vi "ArchViewer.vi"() -> ()   [LabVIEW 2010]
doc: "Use this template to create an application that executes until you click the Stop button. Unlike the Single Loop Application VI that uses polling, this VI uses the Event structure."
uses:
  <vilib>/addons/database/Connection.llb/DB Tools Open Connec (Path).vi
  <vilib>/addons/database/NI_Database_API.lvlib
panel:
  in  "save":bool
  out "Message":string
  out "ObjProp":string[][](table)
  in  "ViewMode":enum32{"Графики", "Тренды/Отчет", "SQL"}(tab)=enum."Тренды/Отчет"
  out "phwnd":string[][](table)
  out "reason":string caption="Описание"
  in  "DateAndTime":u16(ring) caption="Дата и Время" items=["2012-04-04 23:22:02", "2012-05-04 20:10:38"]
  out "Waveform Graph":cluster{sgl, sgl, sgl[]}[](graph)
  in  "CurvesName":i32(ring) caption="Сигнал (Тип сигнала)" items=["Q(wt)max"=400301, "Q(wt)mean"=500301, "Q(R)"=300301, "I(R)"=100301, "N(Q)"=200301]
  in  "DateAndTime 2":u16(ring) caption="Дата и Время" items=["2012-04-04 23:22:02", "2012-05-04 20:10:38"]
  in  "Создать отчет":bool
  out "XY Graph":cluster{timestamp[], sgl[]}(graph)
  in  "T final":timestamp caption="Конец интервала"
  in  "T start":timestamp caption="Начало"
  in  "SigName":u16(ring) caption="Сигнал" items=["Ch1(I(R=0,5))"=2, "Ch1(Q(R=0,5))"=1, "Ch2(I(R=0,5))"=4, "Ch2(Q(R=0,5))"=3, "Ch3(I(R=0,5))"=6, "Ch3(Q(R=0,5))"=5, "Ch4(I(R=0,5))"=8, "Ch4(Q(R=0,5))"=7, "In(Напряжение/Ток)"=10, "In(Частота)"=11, "Out(Напряжение/Ток)"=9]
  in  "Numeric":i32 min=0 max=9
  in  "Execute":bool
  out "Data":string[][](table) caption="Данные"
  in  "Query":string caption="Запрос"
  in  "Tables":i32(listbox) caption="Таблицы"
  in  "Object":u16(ring) caption="Объект" items=["К-19 Тц", "xz_name", "test_5", "object", "object", "xz_name", "object"]
  in  "stop":bool
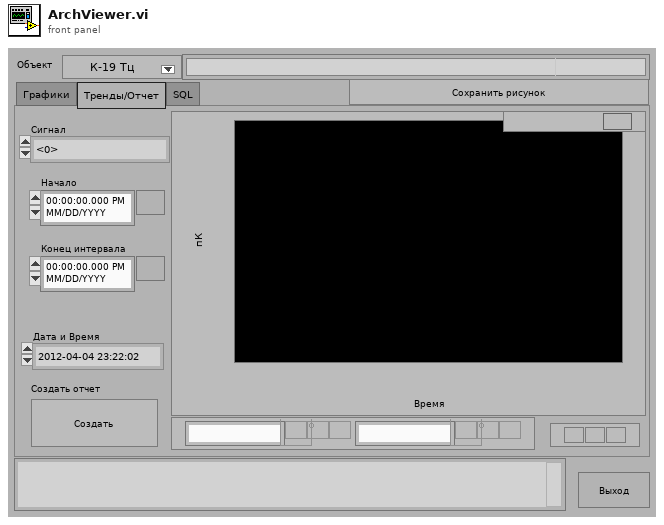
[diagram p1: front panel]
types:
  T1 = cluster{"Number":string, "Obj":string, "SerNum":string, "Graphs":cluster{"Numeric":dbl, "Time Stamp":timestamp, "Array":dbl[]}[]}
  T2 = typedef "NI_Database_API.lvlib/Conn ObjectReference.ctl" = refnum<k1>
  T3 = cluster{"recordset data[0]":variant, "recordset data[1]":variant}
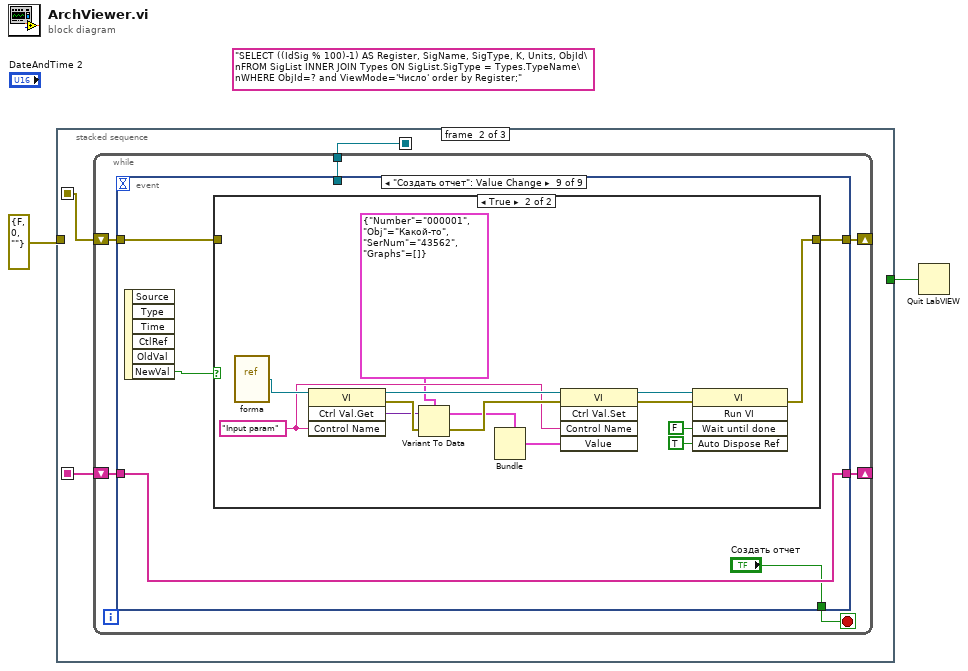
[diagram p0: block diagram]
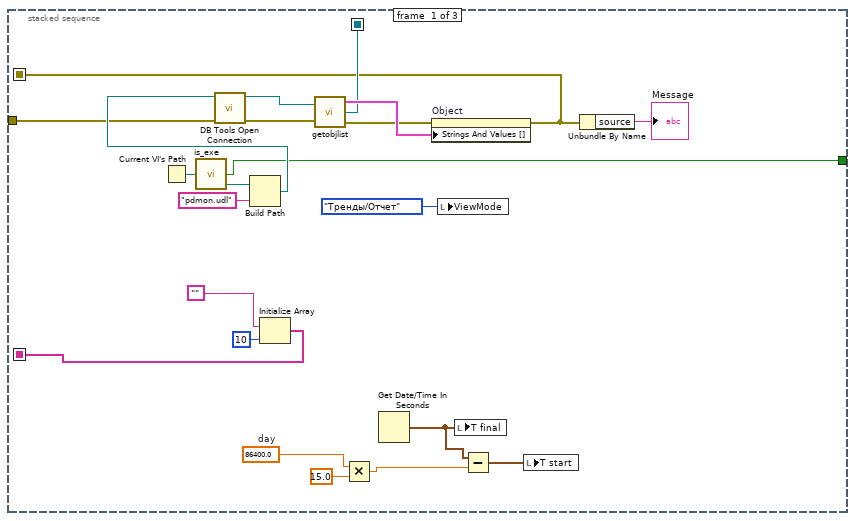
[diagram p2: hidden frame]
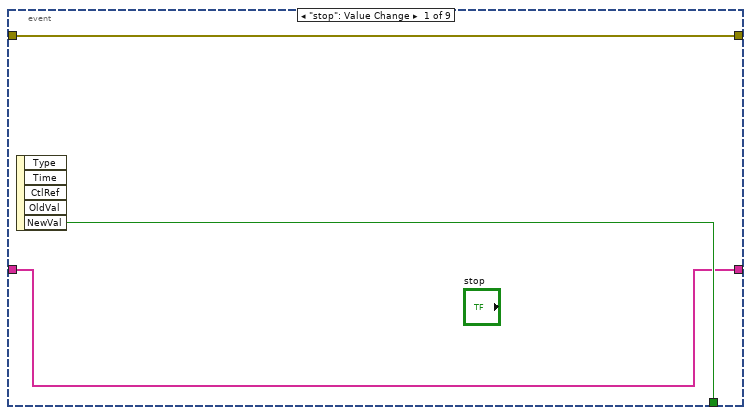
[diagram p3: hidden frame]
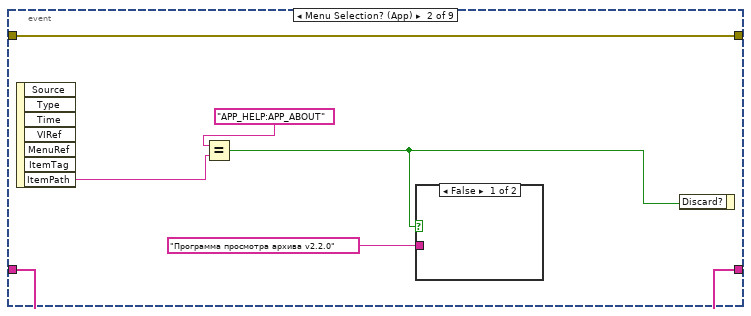
[diagram p4: hidden frame]
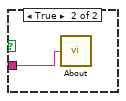
[diagram p5: hidden frame]
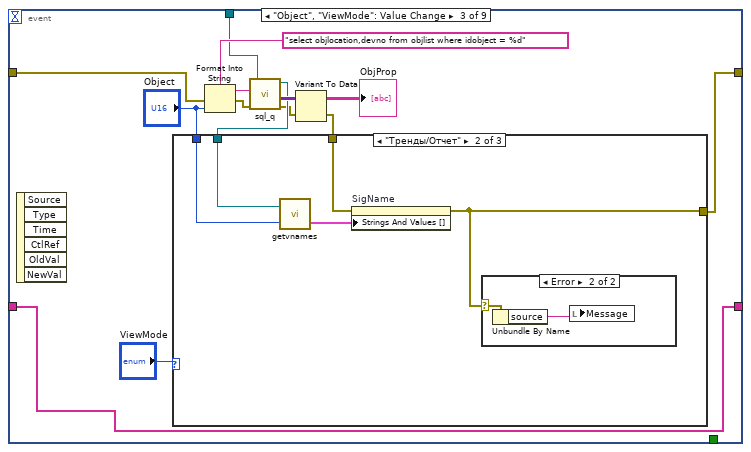
[diagram p6: hidden frame]
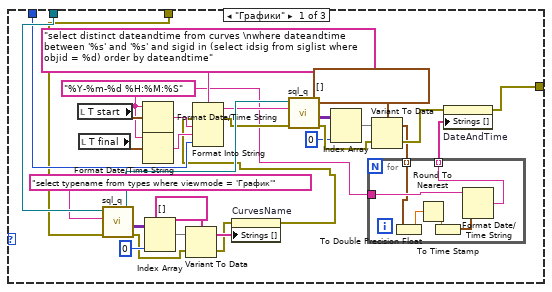
[diagram p7: hidden frame]
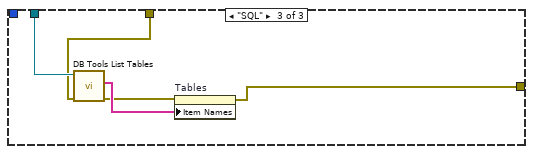
[diagram p9: hidden frame]
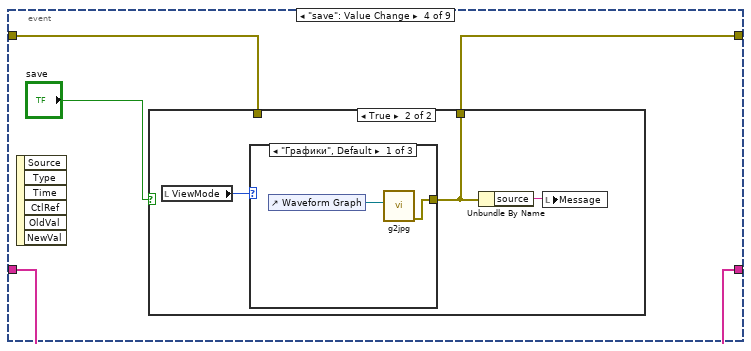
[diagram p10: hidden frame]
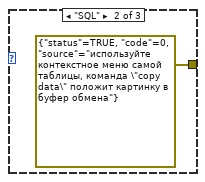
[diagram p12: hidden frame]
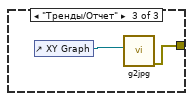
[diagram p13: hidden frame]
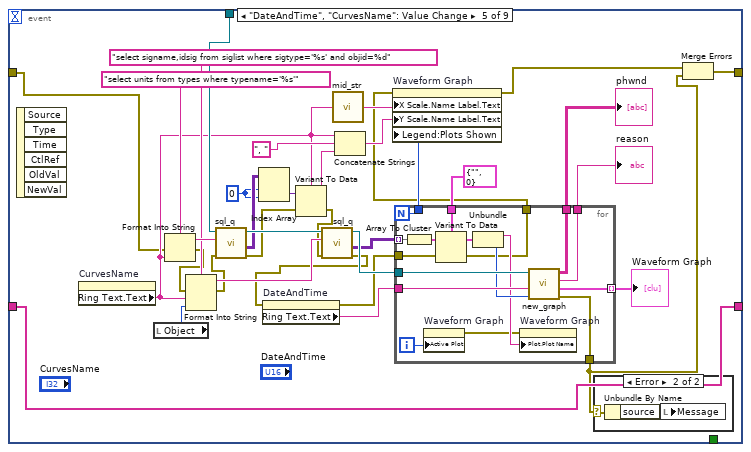
[diagram p14: hidden frame]
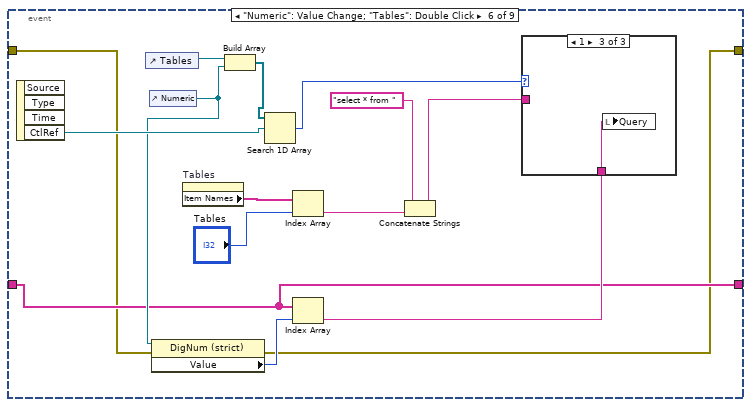
[diagram p16: hidden frame]
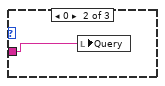
[diagram p18: hidden frame]
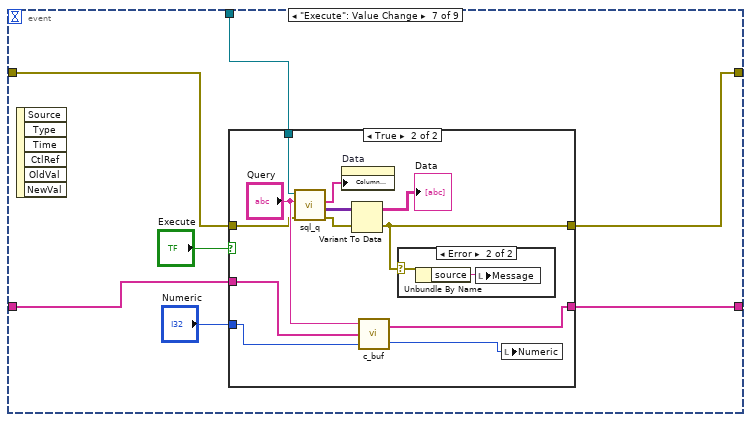
[diagram p19: hidden frame]
diagram:
  (unwired) "SELECT ((IdSig % 100)-1) AS Register, SigName, SigType, K, Units, ObjId\nFROM SigList INNER JOIN Types ON SigList.SigType = Types.TypeName\nWHERE ObjId=? and ViewMode='Число' order by Register;"
  n1 = stacked-sequence {
    seq-local: [w20 _ _] -> [_ w27 w248]
    seq-local: [w7 _ _] -> [_ w26 _]
    seq-local: [w3 _ _] -> [_ w25 _]
    tunnel: [w6 _ _] -> w2
    tunnel: errorcluster {"status"=FALSE, "code"=0, "source"=""} ("error out") -> [w4 _ _]
    frame #0 {
      w12 = 86400.0  # day
      n2 = Current VI's Path() -> (path=w18:path)
      n3 = call "is_exe.vi"("path"=w18) -> ("actual path"=w17:path, "exe?"=w6:bool)  [unwired: 2 in, 1 out]
      n4 = Build Path(base path=w17, name or relative path="pdmon.udl") -> (appended path=w15:path)
      n5 = call-poly <vilib>:"DB Tools Open Connection.vi"("error in (no error)"=w4, "connection information"=w15) -> ("error out"=w21:errorcluster, "connection reference"=w22:T2)  [unwired: 6 in]
      n6 = Initialize Array("", 10 ("dimension size")) -> (w7:string[])
      n7 = call "getobjlist.vi"("connection"=w22, "error in"=w21) -> ("StringsAndValues[]"=w24:cluster{"String":string, "Value":u16}[], "connection out"=w20:T2, "error out"=w23:errorcluster)
      n8 = Multiply(x=w12, y=15.0) -> (x*y=w11:dbl)
      n9 = Get Date/Time In Seconds() -> (seconds since 1Jan1904=w14:timestamp)
      n10 = property on="Object" class="Ring (strict)"(error in=w23, "Strings And Values []"=w24) -> (error out=w3:errorcluster)  [unwired: 1 in, 1 out]
      n11 = local write "ViewMode"(enum32{"Графики", "Тренды/Отчет", "SQL"}."Тренды/Отчет" ("ViewMode")) -> ()
      n12 = local write "T final"(w14) -> ()
      n13 = Subtract(x=w14, y=w11) -> (x-y=w13:timestamp)
      n14 = local write "T start"(w13) -> ()
      n15 = Unbundle By Name(w3) -> ("source"=→"Message":string)
    }
    frame #1 {
      n16 = while {
        tunnel: w27 -> [w32]
        shift-right: [w31] -> _
        shift-left: w26 -> [w30]
        shift-right: [w28] -> _
        shift-left: w25 -> [w29]
        stop <- w33 stop-if-true
        n17 = event shown="[8] \"Создать отчет\": Value Change" {
          selector: _ -> [_ _ _ _ _ _ _ _ _]
          dyn-events: _ -> [_ _ _ _ _ _ _ _ _]
          timeout: _ -> [_ _ _ _ _ _ _ _ _]
          tunnel: [w36 _ _ _ _ _ _ _ "Создать отчет"] -> w33
          tunnel: w32 -> [_ _ w53 _ w142 _ w196 w225 _]
          tunnel: [w35 w42 w47 w108 w130 w175 w193 w218 w232] -> w31
          tunnel: w30 -> [w35 w42 w47 w108 w130 w175 w192 w218 w232]
          tunnel: w29 -> [w34 w37 w46 w106 w126 w174 w191 w216 w231]
          tunnel: [w34 w37 w44 w107 w121 w173 w190 w215 w230] -> w28
          event "stop": Value Change {
            n18 = event-data() -> ("NewVal"=w36:bool)  [unwired: 1 in, 4 out]
          }
          event Menu Selection? (App) {
            n19 = event-data() -> ("ItemPath"=w40:string)  [unwired: 1 in, 6 out]
            n20 = Equal?(x="APP_HELP:APP_ABOUT", y=w40) -> (x = y?=w39:bool)
            n21 = case shown="False" w39 {
              tunnel: "Программа просмотра архива v2.2.0" -> [_ w43]
              frame False {
              }
              frame True {
                n22 = call "About.vi"("Revision Number"=w43) -> ()
              }
            }
            n23 = event-data("Discard?"=w39) -> ()  [unwired: 1 in, 1 out]
          }
          event "Object", "ViewMode": Value Change {
            n24 = event-data() -> ()  [unwired: 1 in, 6 out]
            n25 = Format Into String(format string="select objlocation,devno from objlist where idobject = %d", error in=w46, "Object") -> (resulting string=w56:string, error out=w49:errorcluster)  [unwired: 1 in]
            n26 = call "sql_q.vi"("error in"=w49, "SQL query"=w56, "connect ref"=w53) -> ("error out"=w51:errorcluster, "recordset data"=w55:variant[][], "conn ref out"=w52:T2)  [unwired: 1 in, 1 out]
            n27 = Variant To Data(error in=w51, Variant=w55) -> (error out=w45:errorcluster, data=→"ObjProp":string[][])  [unwired: 1 in]
            n28 = case shown="\"Тренды/Отчет\"" "ViewMode" {
              tunnel: w52 -> [w87 w97 w105]
              tunnel: "Object" -> [w61 w96 _]
              tunnel: w45 -> [w60 w95 w102]
              tunnel: [w58 w94 w101] -> w44
              frame "Графики" {
                w63 = "%Y-%m-%d %H:%M:%S" ("time format string (%c)")
                n29 = local read "T start"() -> (w75:timestamp)
                n30 = local read "T final"() -> (w74:timestamp)
                n31 = call "sql_q.vi"("error in"=w60, "SQL query"="select typename from types where viewmode = 'График'", "connect ref"=w87) -> ("error out"=w80:errorcluster, "recordset data"=w85:variant[][], "conn ref out"=w69:T2)  [unwired: 1 in, 1 out]
                n32 = Format Date/Time String(time format string (%c)=w63, seconds (now)=w75) -> (date/time string=w77:string)  [unwired: 1 in]
                n33 = Format Date/Time String(time format string (%c)=w63, seconds (now)=w74) -> (date/time string=w78:string)  [unwired: 1 in]
                n34 = Index Array(array=w85, index (col)=0 ("disabled index (col)")) -> (element=w82:variant[])  [unwired: 1 in]
                n35 = Variant To Data(error in=w80, Variant=w82, type=string[] [] ("Strings []")) -> (error out=w79:errorcluster, data=w84:string[])
                n36 = property on="CurvesName" class="Ring (strict)"(error in=w79, "Strings []"=w84) -> (error out=w59:errorcluster)  [unwired: 1 in, 1 out]
                n37 = Format Into String(format string="select distinct dateandtime from curves \nwhere dateandtime between '%s' and '%s' and sigid in (select idsig from siglist where objid = %d) order by dateandtime", error in=w59, w77, w78, w61) -> (resulting string=w68:string, error out=w67:errorcluster)  [unwired: 1 in]
                n38 = call "sql_q.vi"("error in"=w67, "SQL query"=w68, "connect ref"=w69) -> ("error out"=w73:errorcluster, "recordset data"=w70:variant[][])  [unwired: 1 in, 2 out]
                n39 = Index Array(array=w70, index (col)=0 ("disabled index (col)")) -> (element=w71:variant[])  [unwired: 1 in]
                n40 = Variant To Data(error in=w73, Variant=w71, type=timestamp[] [] ("Strings []")) -> (error out=w66:errorcluster, data=w65:timestamp[])
                n41 = for {
                  tunnel: w65 -> [w88] mode=indexing
                  tunnel: [w93] -> w64 mode=indexing
                  tunnel: w63 -> [w92]
                  n42 = To Double Precision Float(number=w88) -> (double precision float=w90:dbl)
                  n43 = Round To Nearest(number=w90) -> (nearest integer value=w89:dbl)
                  n44 = To Time Stamp(1:w89) -> (0:w91:timestamp)
                  n45 = Format Date/Time String(time format string (%c)=w92, seconds (now)=w91) -> (date/time string=w93:string)  [unwired: 1 in]
                }
                n46 = property on="DateAndTime" class="Ring (strict)"(error in=w66, "Strings []"=w64) -> (error out=w58:errorcluster)  [unwired: 1 in, 1 out]
              }
              frame "Тренды/Отчет" {
                n47 = call "getvnames.vi"("Object"=w96, "connection reference in"=w97) -> ("StringsAndValues[]"=w98:cluster{"String":string, "Value":u16}[])  [unwired: 1 out]
                n48 = property on="SigName" class="Ring (strict)"(error in=w95, "Strings And Values []"=w98) -> (error out=w94:errorcluster)  [unwired: 1 in, 1 out]
                n49 = case shown="Error" w94 {
                  selector: w94 -> [_ w100]
                  frame No Error {
                  }
                  frame Error {
                    n50 = Unbundle By Name(w100) -> ("source"=w99:string)
                    n51 = local write "Message"(w99) -> ()
                  }
                }
              }
              frame "SQL" {
                n52 = call <vilib>:"DB Tools List Tables.vi"("error in (no error)"=w102, "connection reference"=w105) -> ("error out"=w103:errorcluster, "tables"=w104:string[])  [unwired: 3 in, 1 out]
                n53 = property on="Tables" class="LstBox (strict)"(error in=w103, "Item Names"=w104) -> (error out=w101:errorcluster)  [unwired: 1 in, 1 out]
              }
            }
          }
          event "save": Value Change {
            n54 = event-data() -> ()  [unwired: 1 in, 6 out]
            n55 = case shown="True" "save" {
              tunnel: [w110 w111] -> w107
              tunnel: w106 -> [w110 _]
              frame False {
              }
              frame True {
                n56 = local read "ViewMode"() -> (w113:enum32{"Графики", "Тренды/Отчет", "SQL"})
                n57 = case shown="\"Графики\", Default" w113 {
                  tunnel: [w114 errorcluster {"status"=TRUE, "code"=0, "source"="используйте контекстное меню самой таблицы, команда \"copy data\" положит картинку в буфер обмена"} ("error out") w117] -> w111
                  frame "Графики", Default {
                    n58 = control-ref of="Waveform Graph"() -> (w115:refnum<vi>)
                    n59 = call "g2jpg.vi"("WG"=w115) -> ("error out"=w114:errorcluster)  [unwired: 5 in, 1 out]
                  }
                  frame "SQL" {
                  }
                  frame "Тренды/Отчет" {
                    n60 = control-ref of="XY Graph"() -> (w118:refnum<vi>)
                    n61 = call "g2jpg.vi"("WG"=w118) -> ("error out"=w117:errorcluster)  [unwired: 5 in, 1 out]
                  }
                }
                n62 = Unbundle By Name(w111) -> ("source"=w112:string)
                n63 = local write "Message"(w112) -> ()
              }
            }
          }
          event "DateAndTime", "CurvesName": Value Change {
            w139 = 0
            n64 = event-data() -> ()  [unwired: 1 in, 6 out]
            n65 = property on="CurvesName" class="Ring (strict)"() -> ("Ring Text.Text"=w131:string)  [unwired: 2 in, 2 out]
            n66 = local read "Object"() -> (w150:u16)
            n67 = Format Into String(format string="select units from types where typename='%s'", error in=w126, w131) -> (resulting string=w143:string, error out=w127:errorcluster)  [unwired: 1 in]
            n68 = Format Into String(format string="select signame,idsig from siglist where sigtype='%s' and objid=%d" ("regular expression (\"\")"), error in=w127, w131, w150) -> (resulting string=w151:string, error out=w128:errorcluster)  [unwired: 1 in]
            n69 = call "sql_q.vi"("error in"=w128, "SQL query"=w143, "connect ref"=w142) -> ("error out"=w136:errorcluster, "recordset data"=w140:variant[][], "conn ref out"=w141:T2)  [unwired: 1 in, 1 out]
            n70 = Index Array(array=w140, index (row)=w139, index (col)=w139) -> (element=w138:variant)
            n71 = Variant To Data(error in=w136, Variant=w138, type=w131) -> (error out=w125:errorcluster, data=w135:string)
            n72 = call "sql_q.vi"("error in"=w125, "SQL query"=w151, "connect ref"=w141) -> ("error out"=w120:errorcluster, "recordset data"=w148:variant[][], "conn ref out"=w149:T2)  [unwired: 1 in, 1 out]
            n73 = property on="DateAndTime" class="Ring (strict)"(error in=w120) -> (error out=w119:errorcluster, "Ring Text.Text"=w153:string)  [unwired: 1 in, 1 out]
            n74 = call "mid_str.vi"("String"=w131) -> ("mid substring"=w132:string)  [unwired: 4 in]
            n75 = Concatenate Strings(w131, ", ", w135) -> (w134:string)
            n76 = for {
              N -> [w157]
              tunnel: w153 -> [w170]
              tunnel: [w169] -> w122
              tunnel: [w168] -> w152
              tunnel: w149 -> [w167]
              tunnel: w148 -> [w166] mode=indexing
              tunnel: cluster{string, i32} {"", 0} -> [w165]
              tunnel: [w161] -> w146 mode=indexing
              tunnel: [w157] -> w145
              tunnel: w119 -> [w156]
              tunnel: [w155] -> w124
              tunnel: [w154] -> w129
              i -> [w160]
              n77 = Array To Cluster(array=w166) -> (cluster=w164:T3)
              n78 = property on="Waveform Graph" class="WFGraph (strict)"("Active Plot"=w160) -> (error out=w158:errorcluster)  [unwired: 2 in, 1 out]
              n79 = Variant To Data(error in=w156, Variant=w164, type=w165) -> (error out=w155:errorcluster, data=w163:cluster{string, i32})
              n80 = Unbundle(w163) -> (w159:string, w162:i32)
              n81 = property on="Waveform Graph" class="WFGraph (strict)"(error in=w158, "Plot.Plot Name"=w159) -> ()  [unwired: 1 in, 2 out]
              n82 = call "new_graph.vi"("CurvesId"=w162, "D&T"=w170, "connection ref"=w167) -> ("error out"=w169:errorcluster, "Waveform Graph"=w161:cluster{sgl, sgl, sgl[]}, "reason"=w168:string, "phwnd"=w154:string[][])  [unwired: 1 in]
            }
            "Waveform Graph" <- w146
            "reason" <- w152
            "phwnd" <- w129
            n83 = property on="Waveform Graph" class="WFGraph (strict)"(error in=w124, "X Scale.Name Label.Text"=w132, "Y Scale.Name Label.Text"=w134, "Legend:Plots Shown"=w145) -> (error out=w123:errorcluster)  [unwired: 1 in, 1 out]
            n84 = case shown="Error" w122 {
              selector: w122 -> [_ w172]
              frame No Error {
              }
              frame Error {
                n85 = Unbundle By Name(w172) -> ("source"=w171:string)
                n86 = local write "Message"(w171) -> ()
              }
            }
            n87 = Merge Errors(w123, w122) -> (w121:errorcluster)
          }
          event "Numeric": Value Change; "Tables": Double Click {
            n88 = event-data() -> ("CtlRef"=w181:refnum<vi>)  [unwired: 1 in, 3 out]
            n89 = control-ref of="Tables"() -> (w183:refnum<vi>)
            n90 = control-ref of="Numeric"() -> (w177:refnum<vi>)
            n91 = property on="Property Node" class="DigNum (strict)"(reference=w177, error in=w174) -> (error out=w173:errorcluster, "Value"=w176:i32)  [unwired: 1 out]
            n92 = property on="Tables" class="LstBox (strict)"() -> ("Item Names"=w187:string[])  [unwired: 2 in, 2 out]
            n93 = Build Array(w183, w177) -> (w182:refnum<vi>[])
            n94 = Search 1D Array(1D array=w182, element=w181) -> (index of element=w180:i32)  [unwired: 1 in]
            n95 = Index Array(array=w187, index="Tables") -> (element=w185:string)
            n96 = Index Array(array=w175, index=w176) -> (element=w178:string)
            n97 = Concatenate Strings("select * from " ("format string"), w185) -> (w179:string)
            n98 = case shown="1" w180 {
              tunnel: w179 -> [_ w188 _]
              tunnel: w178 -> [_ _ w189]
              frame -1, Default {
                # "do nothing"
              }
              frame 0 {
                n99 = local write "Query"(w188) -> ()
              }
              frame 1 {
                n100 = local write "Query"(w189) -> ()
              }
            }
          }
          event "Execute": Value Change {
            n101 = event-data() -> ()  [unwired: 1 in, 6 out]
            n102 = case shown="True" "Execute" {
              tunnel: w196 -> [_ w210]
              tunnel: "Numeric" -> [_ w204]
              tunnel: [w198 w205] -> w193
              tunnel: w192 -> [w198 w202]
              tunnel: w191 -> [w197 w200]
              tunnel: [w197 w199] -> w190
              frame False {
              }
              frame True {
                n103 = call "sql_q.vi"("error in"=w200, "SQL query"="Query", "connect ref"=w210) -> ("error out"=w207:errorcluster, "recordset data"=w209:variant[][], "Columns"=w206:string[])  [unwired: 1 in, 1 out]
                n104 = property on="Data" class="Tbl (strict)"("Column Header Strings[]"=w206) -> ()  [unwired: 2 in, 2 out]
                n105 = Variant To Data(error in=w207, Variant=w209) -> (error out=w199:errorcluster, data=→"Data":string[][])  [unwired: 1 in]
                n106 = call "c_buf.vi"("Numeric 2"=w204, "Array"=w202, "Query"="Query") -> ("Numeric"=w203:i32, "Array 2"=w205:string[])
                n107 = case shown="Error" w199 {
                  selector: w199 -> [_ w212]
                  frame No Error {
                  }
                  frame Error {
                    n108 = Unbundle By Name(w212) -> ("source"=w211:string)
                    n109 = local write "Message"(w211) -> ()
                  }
                }
                n110 = local write "Numeric"(w203) -> ()
              }
            }
          }
          event "SigName", "T start", "T final": Value Change {
            n111 = event-data() -> ()  [unwired: 1 in, 6 out]
            n112 = property on="SigName" class="Ring (strict)"(error in=w216) -> (error out=w219:errorcluster, "Ring Text.Text"=w220:string)  [unwired: 1 in, 1 out]
            n113 = call "new_trend.vi"("T start"="T start", "SigId"="SigName", "T final"="T final", "connection ref"=w225) -> ("error out"=w214:errorcluster, "XY Graph"=→"XY Graph":cluster{timestamp[], sgl[]}, "units"=w217:string)  [unwired: 1 out]
            n114 = property on="XY Graph" class="XYGraph (strict)"(error in=w219, "Plot.Plot Name"=w220, "Y Scale.Name Label.Text"=w217) -> (error out=w213:errorcluster)  [unwired: 1 in, 1 out]
            n115 = case shown="Error" w214 {
              selector: w214 -> [_ w227]
              frame No Error {
              }
              frame Error {
                n116 = Unbundle By Name(w227) -> ("source"=w226:string)
                n117 = local write "Message"(w226) -> ()
              }
            }
            n118 = Merge Errors(w213, w214) -> (w215:errorcluster)
          }
          event "Создать отчет": Value Change {
            n119 = event-data() -> ("NewVal"=w228:bool)  [unwired: 1 in, 5 out]
            n120 = case shown="True" w228 {
              tunnel: w231 -> [w233 _]
              tunnel: [w233 w234] -> w230
              frame False {
              }
              frame True {
                w241 = "Input param" ("Control Name")
                n121 = vi-ref "forma.vi"() -> (w242:refnum<vi>)
                n122 = invoke class="VI" method="Ctrl Val.Get"(reference=w242, "Control Name"=w241) -> (reference out=w244:refnum<vi>, error out=w246:errorcluster, "Get Control Value Variant"=w243:variant)  [unwired: 2 in, 1 out]
                n123 = Variant To Data(error in=w246, Variant=w243, type=T1 {"Number"="000001", "Obj"="Какой-то", "SerNum"="43562", "Graphs"=[]} ("Input param")) -> (error out=w247:errorcluster, data=w240:T1)
                n124 = Bundle(cluster=w240) -> (w245:T1)  [unwired: 4 in]
                n125 = invoke class="VI" method="Ctrl Val.Set"(reference=w244, error in=w247, "Control Name"=w241, "Value"=w245) -> (reference out=w238:refnum<vi>, error out=w235:errorcluster)  [unwired: 1 in, 3 out]
                n126 = invoke class="VI" method="Run VI"(reference=w238, error in=w235, "Wait until done"=FALSE ("Wait Until Done"), "Auto Dispose Ref"=TRUE ("Auto Dispose Reference")) -> (error out=w234:errorcluster)  [unwired: 1 in, 4 out]
              }
            }
          }
        }
      }
    }
    frame #2 {
      n127 = call <vilib>:"DB Tools Close Connection.vi"("connection reference"=w248) -> ()  [unwired: 6 in, 1 out]
    }
  }
  n128 = Quit LabVIEW(quit? (T)=w2) -> ()
